vi "黑盾空调.vi"() -> ()   [LabVIEW 2016, in "环境动力监测库.lvlib" / "空调库.lvlib"]
uses:
  <vilib>/Utility/config.llb/NI_LVConfig.lvlib
  <vilib>/ptbypt/NI_PtbyPt.lvlib
panel:
  out "串口":string
  out "传感器状态":T1 {"系统模拟量量化数据"."电流A" format="%#.2g"}
  in  "查看型号":bool
  in  "重开串口":bool
  in  "校时":bool
  in  "设定参数":bool
  in  "遥控":bool
  out "获取设备厂家信息":T2
  out "仪器时间":timestamp
  out "系统参数":T3
  out "告警状态":T4
  out "写入缓冲区":string
  out "读取缓冲区":string
  out "读取选择":string(combo)
  out "通讯":bool
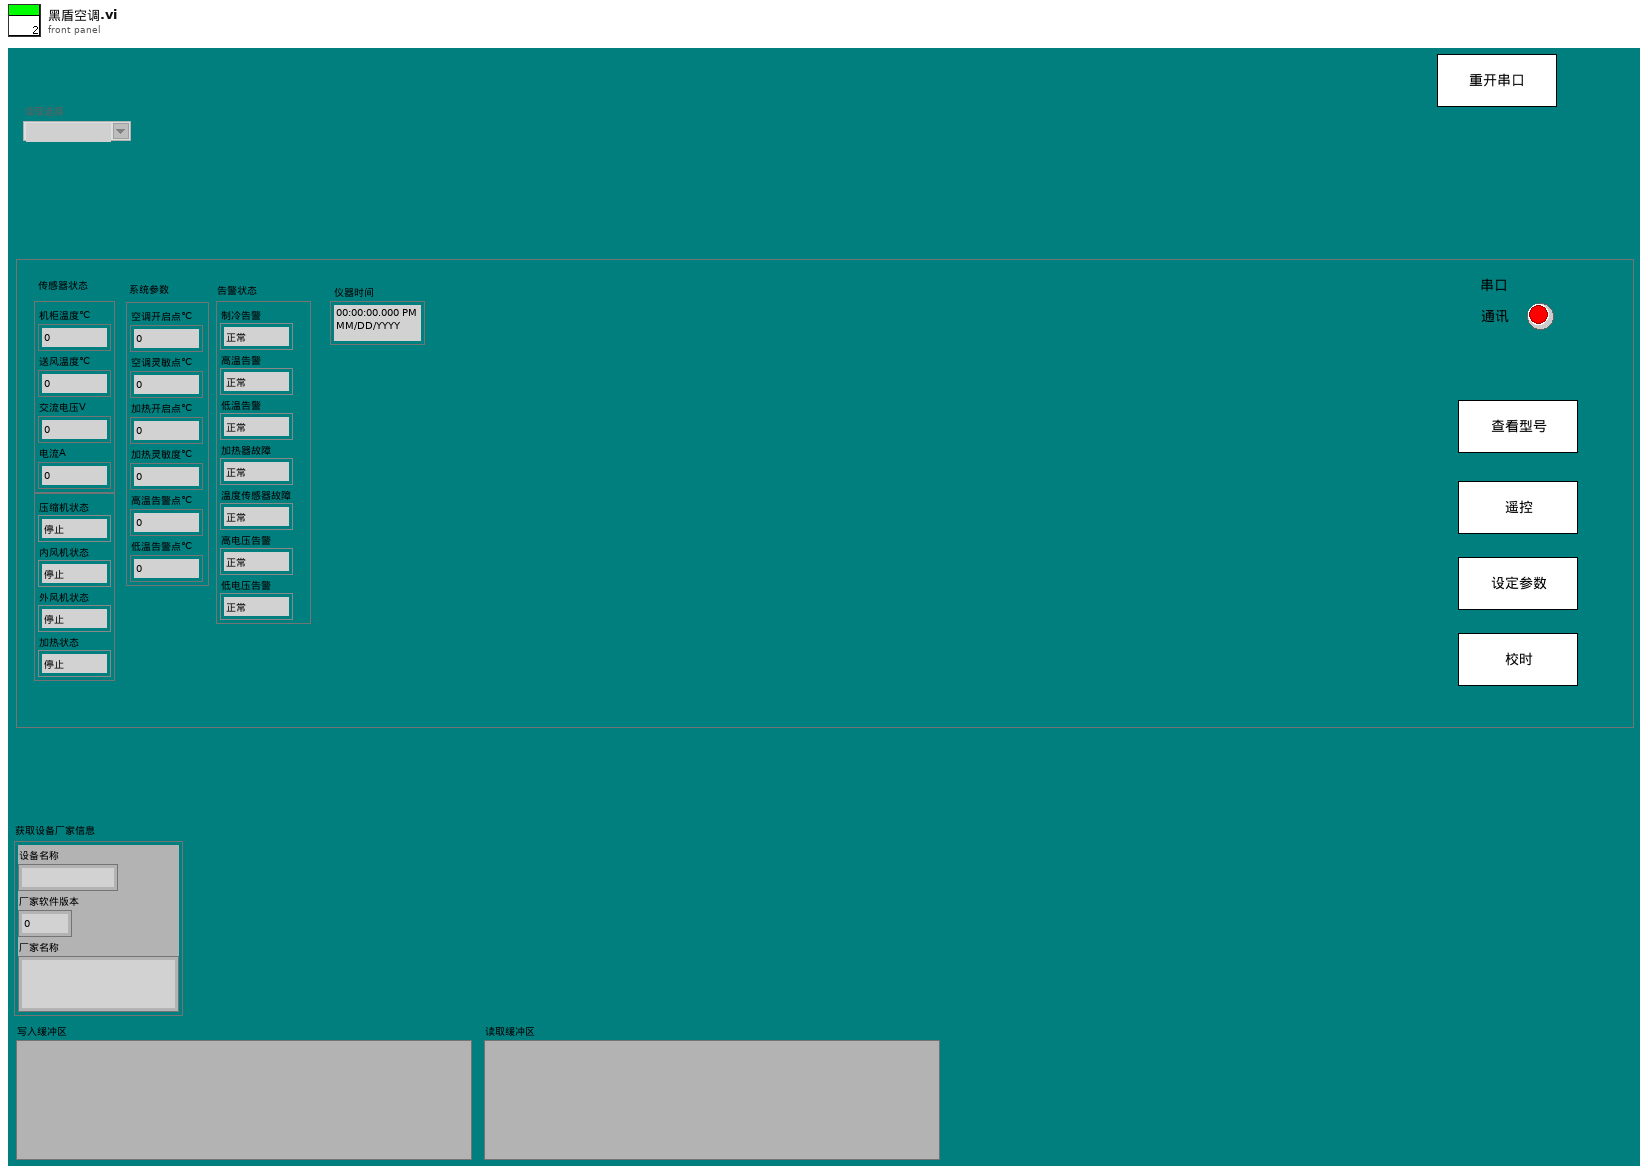
[diagram p1: front panel]
types:
  T1 = cluster{"系统模拟量量化数据":cluster{"机柜温度℃":sgl, "送风温度℃":sgl, "交流电压V":sgl, "电流A":sgl}, "开关量输入状态解析":cluster{"压缩机状态":enum16{"停止", "运行"}, "内风机状态":enum16{"停止", "运行"}, "外风机状态":enum16{"停止", "运行"}, "加热状态":enum16{"停止", "运行"}}}
  T2 = cluster{"设备名称":string, "厂家软件版本":u16, "厂家名称":string}
  T3 = cluster{"空调开启点℃":u16, "空调灵敏点℃":u16, "加热开启点℃":u16, "加热灵敏度℃":u16, "高温告警点℃":u16, "低温告警点℃":u16}
  T4 = cluster{"制冷告警":enum16{"正常", "告警"}, "高温告警":enum16{"正常", "告警"}, "低温告警":enum16{"正常", "告警"}, "加热器故障":enum16{"正常", "告警"}, "温度传感器故障":enum16{"正常", "告警"}, "高电压告警":enum16{"正常", "告警"}, "低电压告警":enum16{"正常", "告警"}, "预留":u16}
  T5 = cluster{"分支":enum16{"open", "read", "write", "close"}, "字符串":string}
  T6 = cluster{"分支":enum16{"open", "read", "write", "close"}, "读取选择":string}
  T7 = typedef "NI_LVConfig.lvlib/Config Data RefNum.ctl" = refnum<k1>
  T8 = cluster{"时间标识":timestamp, "设备":string, "日志信息":string}
  T9 = cluster{"漏水监测输出":cluster{"漏水监测告警":bool, "告警内容":string}, "门禁监测输出":cluster{"门禁监测告警":bool, "告警内容":string}, "温湿度监测输出":cluster{"温湿度监测告警":bool, "告警内容":string}, "烟雾监测输出":cluster{"烟雾监测告警":bool, "告警内容":string}, "空调监测输出":cluster{"空调监测告警":bool, "告警内容":string}, "自动重合闸输出":cluster{"自动重合闸告警":bool, "告警内容":string}, "红外入侵输出":cluster{"红外入侵告警":bool, "告警内容":string}, "振动输出":cluster{"振动告警":bool, "告警内容":string}, "UPS输出":cluster{"UPS告警":bool, "告警内容":string}, "蓄电池输出":cluster{"蓄电池告警":bool, "告警内容":string}, "GPS输出":cluster{"定位告警":bool, "告警内容":string}, "北斗输出":cluster{"定位告警":bool, "告警内容":string}, "气象输出":cluster{"气象告警":bool, "告警内容":string}}
  T10 = cluster{"温湿度":cluster{"温度:":sgl, "状态":bool, "湿度:":sgl}, "空调":cluster{"机柜温度:":sgl, "状态":bool, "压缩机:":enum16{"停止", "运行"}, "电加热:":enum16{"停止", "运行"}}, "排气扇":cluster{"排气扇:":enum16{"关闭", "打开"}}, "冰箱":cluster{"冰箱:":enum16{"关闭", "打开"}}}
  T11 = enum16{"获取模拟量量化数据（浮点数）", "获取模拟量量化数据（定点数）", "获取开关输入状态", "获取机柜空调告警状态", "遥控", "获取系统参数（浮点数）", "获取系统参数（定点数）", "设定系统参数（浮点数）", "设定系统参数（定点数）", "获取系统历史数据（浮点数）", "获取系统历史数据（定点数）", "获取历史告警", "获取监测模块时间", "设定监测模块时间", "获取通信协议版本号", "获取设备地址", "获取设备厂家信息", "设定设备地址（ADR）"}
  T12 = cluster{"分支":enum16{"open", "read", "write", "close"}, "连接的字符串":string}
  T13 = cluster{"机柜温度":sgl, "送风温度":sgl, "交流电压":sgl, "电流":sgl}
  T14 = cluster{"空调状态":enum16{"停止", "运行"}, "内风机状态":enum16{"停止", "运行"}, "外风机状态":enum16{"停止", "运行"}, "加热状态":enum16{"停止", "运行"}}
  T15 = cluster{"空调开启点":u16, "空调灵敏点":u16, "加热开启点":u16, "加热灵敏度":u16, "高温告警点":u16, "低温告警点":u16}
  T16 = enum16{"空调开机", "空调关机", "制冷开启", "制冷关闭", "制热开启", "制热关闭"}
  T17 = enum16{"空调开启点", "空调灵敏点", "加热开启点", "加热灵敏度", "高温告警点", "低温告警点"}
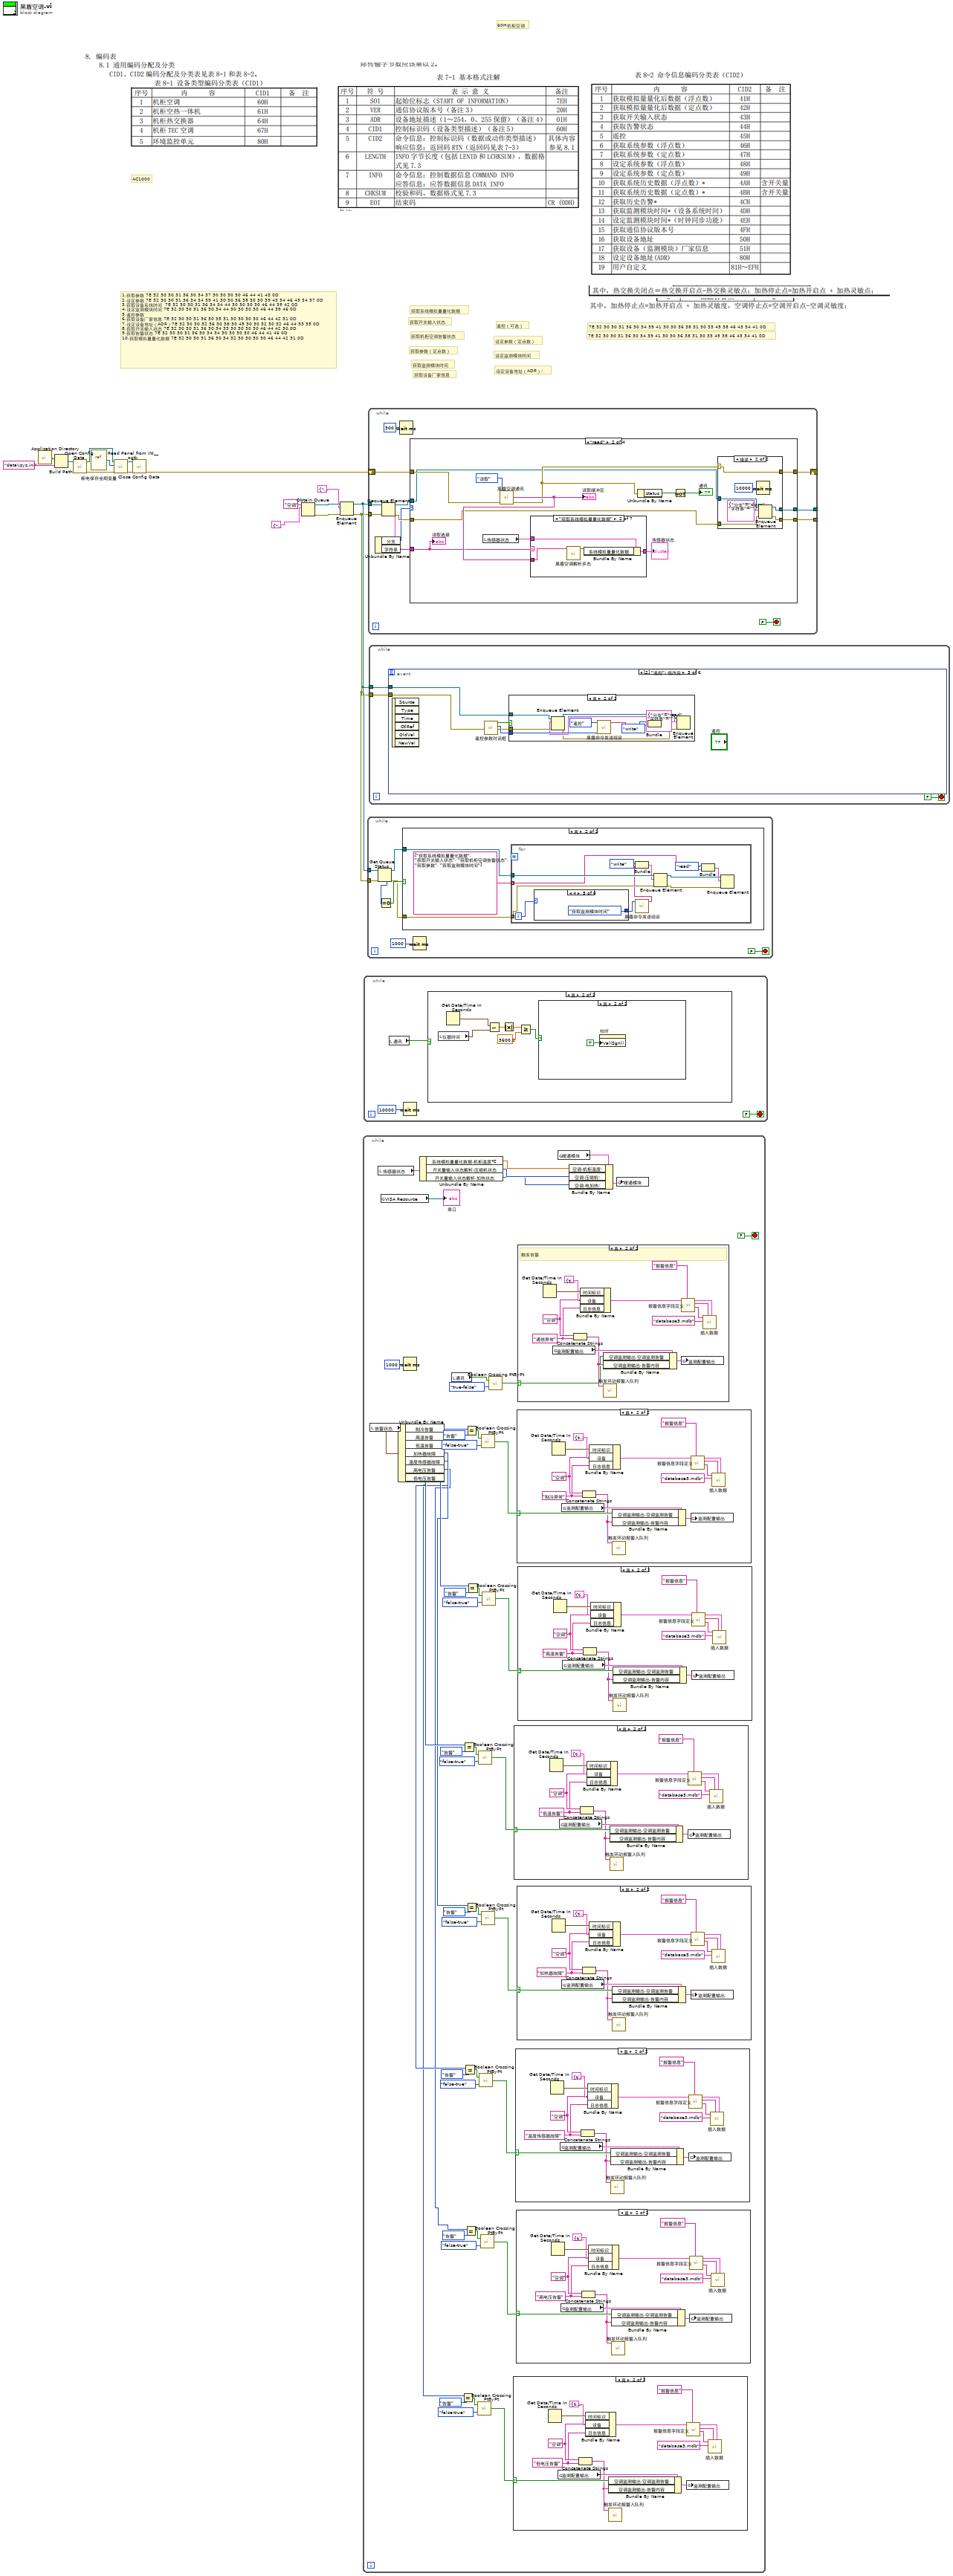
[diagram p0: block diagram]
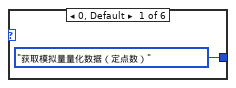
[diagram p13: hidden frame]
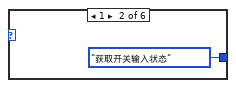
[diagram p14: hidden frame]
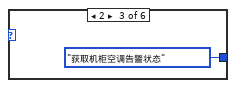
[diagram p15: hidden frame]
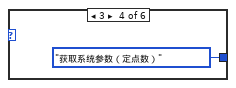
[diagram p16: hidden frame]
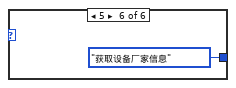
[diagram p17: hidden frame]
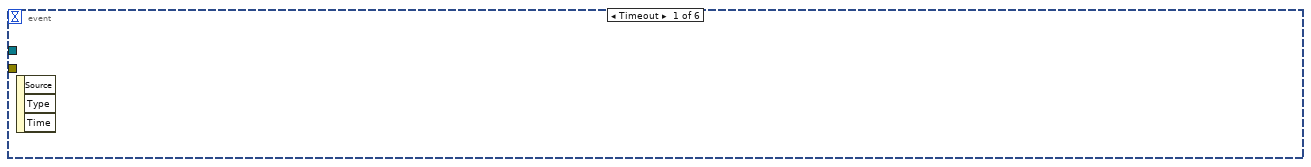
[diagram p18: hidden frame]
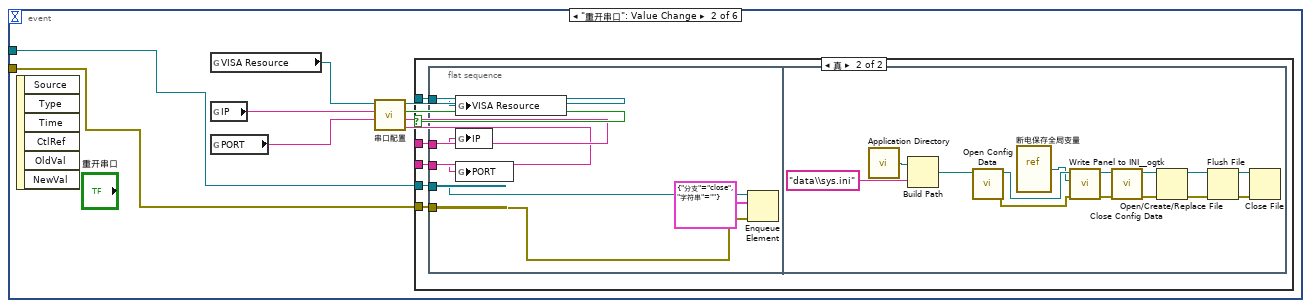
[diagram p19: hidden frame]
diagram:
  # "获取系统模拟量量化数据"
  # "设定设备地址（ADR）:"
  # "获取设备厂家信息"
  # "设定监测模块时间"
  # "获取监测模块时间"
  # "设定参数（定点数）"
  # "获取参数（定点数）"
  # "遥控（可选）"
  # "获取机柜空调告警状态"
  # "获取开关输入状态"
  # "7E 32 30 30 31 36 30 34 39 41 30 30 36 38 31 30 33 45 38 46 43 34 41 0D"
  # "7E 32 30 30 31 36 30 34 39 41 30 30 36 38 31 30 33 45 38 46 43 34 41 0D"
  # "60H机柜空调"
  # "AC1000"
  # "1.获取参数 7E 32 30 30 31 36 30 34 37 30 30 30 30 46 44 41 43 0D\n2.设定参数 7E 32 30 30 31 36 34 34 39 41 30 30 36 38 30 30 39 43 34 46 43 34 37 0D \n3.获取设备系统时间  7E 32 30 30 31 36 34 34 44 30 30 30 30 46 44 39 42 0D\n4.设定监测模块时间 7E 32 30 30 31 36 30 34 44 30 30 30 30 46 44 39 46 0D\n5.遥控参数\n6.获取设备厂家信息 7E 32 30 30 31 36 30 35 31 30 30 30 30 46 44 42 31 0D\n7.设定设备地址（ADR）7E 32 30 30 32 36 30 38 30 45 30 30 32 30 32 46 44 33 35 0D\n8.获取开关输入状态 7E 32 30 30 31 36 30 34 33 30 30 30 30 46 44 42 30 0D\n9.获取告警状态 7E 32 30 30 31 36 30 34 34 30 30 30 30 46 44 41 46 0D\n10.获取模拟量量化数据 7E 32 30 30 31 36 30 34 32 30 30 30 30 46 44 42 31 0D"
  n1 = call <vilib>:"Application Directory.vi"() -> ("Application Directory"=w16:path)
  n2 = Build Path(base path=w16, name or relative path="data\\sys.ini" ("名称或相对路径")) -> (appended path=w14:path)
  n3 = call <vilib>:"Open Config Data.vi"("configuration file path"=w14) -> ("error out"=w10:errorcluster, "refnum"=w13:T7)  [unwired: 8 in, 1 out]
  n4 = vi-ref "断电保存全局变量.vi"() -> (w12:refnum<vi>)
  n5 = call <userlib>:"Read Panel from INI__ogtk.vi"("error in (no error)"=w10, "VI ref"=w12, "refnum"=w13) -> ("error out"=w9:errorcluster, "refnum out"=w11:T7)  [unwired: 7 in]
  n6 = call <vilib>:"Close Config Data.vi"("error in (no error)"=w9, "refnum"=w11) -> ("error out"=w8:errorcluster)  [unwired: 8 in, 1 out]
  n7 = Obtain Queue(name (unnamed)="空调" ("名称（未命名）"), element data type=T5 {"分支"=enum."open", "字符串"="获取系统模拟量量化数据"}) -> (queue out=w6:refnum<queue>, error out=w5:errorcluster)  [unwired: 3 in, 1 out]
  n8 = Enqueue Element(queue=w6, element=T6 {"分支"=enum."open", "读取选择"="获取系统模拟量量化数据"}, error in (no error)=w5) -> (queue out=w4:refnum<queue>, error out=w3:errorcluster)  [unwired: 1 in, 1 out]
  n9 = while {
    stop <- FALSE stop-if-true
    n10 = local read "告警状态"() -> (w52:T4)
    n11 = local read "传感器状态"() -> (w59:T1)
    n12 = global read "断电保存全局变量.vi" "VISA Resource"() -> (→"串口":refnum<visa-resource-name>)
    n13 = Unbundle By Name(w52) -> ("制冷告警"=w51:enum16{"正常", "告警"}, "高温告警"=w42:enum16{"正常", "告警"}, "低温告警"=w37:enum16{"正常", "告警"}, "加热器故障"=w32:enum16{"正常", "告警"}, "温度传感器故障"=w27:enum16{"正常", "告警"}, "高电压告警"=w18:enum16{"正常", "告警"}, "低电压告警"=w17:enum16{"正常", "告警"})
    n14 = Wait (ms)(milliseconds to wait=u32 1000 ("等待时间（毫秒）")) -> ()  [unwired: 1 out]
    n15 = Unbundle By Name(w59) -> ("系统模拟量量化数据.机柜温度℃"=w58:sgl, "开关量输入状态解析.压缩机状态"=w57:enum16{"停止", "运行"}, "开关量输入状态解析.加热状态"=w56:enum16{"停止", "运行"})
    n16 = local read "通讯"() -> (w53:bool)
    n17 = Equal?(x=w17, y=enum16{"正常", "告警"}."告警") -> (x = y?=w20:bool)
    n18 = Equal?(x=w37, y=enum16{"正常", "告警"}."告警") -> (x = y?=w39:bool)
    n19 = Equal?(x=w27, y=enum16{"正常", "告警"}."告警") -> (x = y?=w29:bool)
    n20 = Equal?(x=w18, y=enum16{"正常", "告警"}."告警") -> (x = y?=w24:bool)
    n21 = Equal?(x=w51, y=enum16{"正常", "告警"}."告警") -> (x = y?=w48:bool)
    n22 = Equal?(x=w32, y=enum16{"正常", "告警"}."告警") -> (x = y?=w34:bool)
    n23 = Equal?(x=w42, y=enum16{"正常", "告警"}."告警") -> (x = y?=w44:bool)
    n24 = call <vilib>:"Boolean Crossing PtByPt.vi"("direction"=enum16{"either", "false-true", "true-false"}."false-true", "input"=w20) -> ("crossing"=w19:bool)  [unwired: 1 in]
    n25 = call <vilib>:"Boolean Crossing PtByPt.vi"("direction"=enum16{"either", "false-true", "true-false"}."false-true", "input"=w39) -> ("crossing"=w38:bool)  [unwired: 1 in]
    n26 = call <vilib>:"Boolean Crossing PtByPt.vi"("direction"=enum16{"either", "false-true", "true-false"}."false-true", "input"=w29) -> ("crossing"=w28:bool)  [unwired: 1 in]
    n27 = call <vilib>:"Boolean Crossing PtByPt.vi"("direction"=enum16{"either", "false-true", "true-false"}."false-true", "input"=w24) -> ("crossing"=w23:bool)  [unwired: 1 in]
    n28 = call <vilib>:"Boolean Crossing PtByPt.vi"("direction"=enum16{"either", "false-true", "true-false"}."false-true", "input"=w48) -> ("crossing"=w47:bool)  [unwired: 1 in]
    n29 = call <vilib>:"Boolean Crossing PtByPt.vi"("direction"=enum16{"either", "false-true", "true-false"}."false-true", "input"=w34) -> ("crossing"=w33:bool)  [unwired: 1 in]
    n30 = call <vilib>:"Boolean Crossing PtByPt.vi"("direction"=enum16{"either", "false-true", "true-false"}."false-true", "input"=w44) -> ("crossing"=w43:bool)  [unwired: 1 in]
    n31 = call <vilib>:"Boolean Crossing PtByPt.vi"("direction"=enum16{"either", "false-true", "true-false"}."true-false", "input"=w53) -> ("crossing"=w54:bool)  [unwired: 1 in]
    n32 = case shown="真" w19 {
      selector: w19 -> [_ w68]
      frame False {
      }
      frame True {
        w66 = "低电压告警" ("日志信息")
        w67 = "空调" ("设备")
        n33 = Get Date/Time In Seconds() -> (seconds since 1Jan1904=w78:timestamp)
        n34 = global read "断电保存全局变量.vi" "监测配置输出"() -> (w69:T9)
        n35 = Concatenate Strings(w67, w66) -> (w65:string)
        n36 = Bundle By Name(cluster=T8 {"时间标识"=timestamp(0 s since 1904-01-01), "设备"="", "日志信息"=""} ("data in"), "时间标识"=w78, "设备"=w67, "日志信息"=w66) -> (w77:T8)
        n37 = Bundle By Name(cluster=w69, "空调监测输出.空调监测告警"=w68, "空调监测输出.告警内容"=w65) -> (w70:T9)
        n38 = call "触发环动报警入队列.vi"("报警内容"=w65) -> ()  [unwired: 11 in]
        n39 = call "报警信息字段定义.vi"("table输入"="报警信息", "data in"=w77) -> ("table输出"=w73:string, "columns"=w72:string[], "data out"=w71:T8)  [unwired: 7 in]
        n40 = global write "断电保存全局变量.vi" "监测配置输出"(w70) -> ()
        n41 = call "插入数据.vi"("data"=w71, "columns"=w72, "database"="database3.mdb", "table"=w73) -> ()  [unwired: 7 in, 1 out]
      }
    }
    n42 = case shown="真" w38 {
      selector: w38 -> [_ w124]
      frame False {
      }
      frame True {
        w122 = "低温告警" ("日志信息")
        w123 = "空调" ("设备")
        n43 = Get Date/Time In Seconds() -> (seconds since 1Jan1904=w134:timestamp)
        n44 = global read "断电保存全局变量.vi" "监测配置输出"() -> (w125:T9)
        n45 = Concatenate Strings(w123, w122) -> (w121:string)
        n46 = Bundle By Name(cluster=T8 {"时间标识"=timestamp(0 s since 1904-01-01), "设备"="", "日志信息"=""} ("data in"), "时间标识"=w134, "设备"=w123, "日志信息"=w122) -> (w133:T8)
        n47 = Bundle By Name(cluster=w125, "空调监测输出.空调监测告警"=w124, "空调监测输出.告警内容"=w121) -> (w126:T9)
        n48 = call "触发环动报警入队列.vi"("报警内容"=w121) -> ()  [unwired: 11 in]
        n49 = call "报警信息字段定义.vi"("table输入"="报警信息", "data in"=w133) -> ("table输出"=w129:string, "columns"=w128:string[], "data out"=w127:T8)  [unwired: 7 in]
        n50 = global write "断电保存全局变量.vi" "监测配置输出"(w126) -> ()
        n51 = call "插入数据.vi"("data"=w127, "columns"=w128, "database"="database3.mdb", "table"=w129) -> ()  [unwired: 7 in, 1 out]
      }
    }
    n52 = case shown="真" w28 {
      selector: w28 -> [_ w96]
      frame False {
      }
      frame True {
        w94 = "温度传感器故障" ("日志信息")
        w95 = "空调" ("设备")
        n53 = Get Date/Time In Seconds() -> (seconds since 1Jan1904=w106:timestamp)
        n54 = global read "断电保存全局变量.vi" "监测配置输出"() -> (w97:T9)
        n55 = Concatenate Strings(w95, w94) -> (w93:string)
        n56 = Bundle By Name(cluster=T8 {"时间标识"=timestamp(0 s since 1904-01-01), "设备"="", "日志信息"=""} ("data in"), "时间标识"=w106, "设备"=w95, "日志信息"=w94) -> (w105:T8)
        n57 = Bundle By Name(cluster=w97, "空调监测输出.空调监测告警"=w96, "空调监测输出.告警内容"=w93) -> (w98:T9)
        n58 = call "触发环动报警入队列.vi"("报警内容"=w93) -> ()  [unwired: 11 in]
        n59 = call "报警信息字段定义.vi"("table输入"="报警信息", "data in"=w105) -> ("table输出"=w101:string, "columns"=w100:string[], "data out"=w99:T8)  [unwired: 7 in]
        n60 = global write "断电保存全局变量.vi" "监测配置输出"(w98) -> ()
        n61 = call "插入数据.vi"("data"=w99, "columns"=w100, "database"="database3.mdb", "table"=w101) -> ()  [unwired: 7 in, 1 out]
      }
    }
    n62 = case shown="真" w23 {
      selector: w23 -> [_ w82]
      frame False {
      }
      frame True {
        w80 = "高电压告警" ("日志信息")
        w81 = "空调" ("设备")
        n63 = Get Date/Time In Seconds() -> (seconds since 1Jan1904=w92:timestamp)
        n64 = global read "断电保存全局变量.vi" "监测配置输出"() -> (w83:T9)
        n65 = Concatenate Strings(w81, w80) -> (w79:string)
        n66 = Bundle By Name(cluster=T8 {"时间标识"=timestamp(0 s since 1904-01-01), "设备"="", "日志信息"=""} ("data in"), "时间标识"=w92, "设备"=w81, "日志信息"=w80) -> (w91:T8)
        n67 = Bundle By Name(cluster=w83, "空调监测输出.空调监测告警"=w82, "空调监测输出.告警内容"=w79) -> (w84:T9)
        n68 = call "触发环动报警入队列.vi"("报警内容"=w79) -> ()  [unwired: 11 in]
        n69 = call "报警信息字段定义.vi"("table输入"="报警信息", "data in"=w91) -> ("table输出"=w87:string, "columns"=w86:string[], "data out"=w85:T8)  [unwired: 7 in]
        n70 = global write "断电保存全局变量.vi" "监测配置输出"(w84) -> ()
        n71 = call "插入数据.vi"("data"=w85, "columns"=w86, "database"="database3.mdb", "table"=w87) -> ()  [unwired: 7 in, 1 out]
      }
    }
    n72 = case shown="真" w47 {
      selector: w47 -> [_ w152]
      frame False {
      }
      frame True {
        w150 = "制冷异常" ("日志信息")
        w151 = "空调" ("设备")
        n73 = Get Date/Time In Seconds() -> (seconds since 1Jan1904=w162:timestamp)
        n74 = global read "断电保存全局变量.vi" "监测配置输出"() -> (w153:T9)
        n75 = Concatenate Strings(w151, w150) -> (w149:string)
        n76 = Bundle By Name(cluster=T8 {"时间标识"=timestamp(0 s since 1904-01-01), "设备"="", "日志信息"=""} ("data in"), "时间标识"=w162, "设备"=w151, "日志信息"=w150) -> (w161:T8)
        n77 = Bundle By Name(cluster=w153, "空调监测输出.空调监测告警"=w152, "空调监测输出.告警内容"=w149) -> (w154:T9)
        n78 = call "触发环动报警入队列.vi"("报警内容"=w149) -> ()  [unwired: 11 in]
        n79 = call "报警信息字段定义.vi"("table输入"="报警信息", "data in"=w161) -> ("table输出"=w157:string, "columns"=w156:string[], "data out"=w155:T8)  [unwired: 7 in]
        n80 = global write "断电保存全局变量.vi" "监测配置输出"(w154) -> ()
        n81 = call "插入数据.vi"("data"=w155, "columns"=w156, "database"="database3.mdb", "table"=w157) -> ()  [unwired: 7 in, 1 out]
      }
    }
    n82 = case shown="真" w33 {
      selector: w33 -> [_ w110]
      frame False {
      }
      frame True {
        w108 = "加热器故障" ("日志信息")
        w109 = "空调" ("设备")
        n83 = Get Date/Time In Seconds() -> (seconds since 1Jan1904=w120:timestamp)
        n84 = global read "断电保存全局变量.vi" "监测配置输出"() -> (w111:T9)
        n85 = Concatenate Strings(w109, w108) -> (w107:string)
        n86 = Bundle By Name(cluster=T8 {"时间标识"=timestamp(0 s since 1904-01-01), "设备"="", "日志信息"=""} ("data in"), "时间标识"=w120, "设备"=w109, "日志信息"=w108) -> (w119:T8)
        n87 = Bundle By Name(cluster=w111, "空调监测输出.空调监测告警"=w110, "空调监测输出.告警内容"=w107) -> (w112:T9)
        n88 = call "触发环动报警入队列.vi"("报警内容"=w107) -> ()  [unwired: 11 in]
        n89 = call "报警信息字段定义.vi"("table输入"="报警信息", "data in"=w119) -> ("table输出"=w115:string, "columns"=w114:string[], "data out"=w113:T8)  [unwired: 7 in]
        n90 = global write "断电保存全局变量.vi" "监测配置输出"(w112) -> ()
        n91 = call "插入数据.vi"("data"=w113, "columns"=w114, "database"="database3.mdb", "table"=w115) -> ()  [unwired: 7 in, 1 out]
      }
    }
    n92 = case shown="真" w54 {
      selector: w54 -> [_ w163]
      frame False {
      }
      frame True {
        w165 = "通信异常" ("日志信息")
        w166 = "空调" ("设备")
        # "触发告警"
        n93 = Get Date/Time In Seconds() -> (seconds since 1Jan1904=w176:timestamp)
        n94 = global read "断电保存全局变量.vi" "监测配置输出"() -> (w167:T9)
        n95 = Concatenate Strings(w166, w165) -> (w164:string)
        n96 = Bundle By Name(cluster=T8 {"时间标识"=timestamp(0 s since 1904-01-01), "设备"="", "日志信息"=""} ("data in"), "时间标识"=w176, "设备"=w166, "日志信息"=w165) -> (w175:T8)
        n97 = Bundle By Name(cluster=w167, "空调监测输出.空调监测告警"=w163, "空调监测输出.告警内容"=w164) -> (w168:T9)
        n98 = call "触发环动报警入队列.vi"("报警内容"=w164) -> ()  [unwired: 11 in]
        n99 = call "报警信息字段定义.vi"("table输入"="报警信息", "data in"=w175) -> ("table输出"=w171:string, "columns"=w170:string[], "data out"=w169:T8)  [unwired: 7 in]
        n100 = global write "断电保存全局变量.vi" "监测配置输出"(w168) -> ()
        n101 = call "插入数据.vi"("data"=w169, "columns"=w170, "database"="database3.mdb", "table"=w171) -> ()  [unwired: 7 in, 1 out]
      }
    }
    n102 = case shown="真" w43 {
      selector: w43 -> [_ w138]
      frame False {
      }
      frame True {
        w136 = "高温告警" ("日志信息")
        w137 = "空调" ("设备")
        n103 = Get Date/Time In Seconds() -> (seconds since 1Jan1904=w148:timestamp)
        n104 = global read "断电保存全局变量.vi" "监测配置输出"() -> (w139:T9)
        n105 = Concatenate Strings(w137, w136) -> (w135:string)
        n106 = Bundle By Name(cluster=T8 {"时间标识"=timestamp(0 s since 1904-01-01), "设备"="", "日志信息"=""} ("data in"), "时间标识"=w148, "设备"=w137, "日志信息"=w136) -> (w147:T8)
        n107 = Bundle By Name(cluster=w139, "空调监测输出.空调监测告警"=w138, "空调监测输出.告警内容"=w135) -> (w140:T9)
        n108 = call "触发环动报警入队列.vi"("报警内容"=w135) -> ()  [unwired: 11 in]
        n109 = call "报警信息字段定义.vi"("table输入"="报警信息", "data in"=w147) -> ("table输出"=w143:string, "columns"=w142:string[], "data out"=w141:T8)  [unwired: 7 in]
        n110 = global write "断电保存全局变量.vi" "监测配置输出"(w140) -> ()
        n111 = call "插入数据.vi"("data"=w141, "columns"=w142, "database"="database3.mdb", "table"=w143) -> ()  [unwired: 7 in, 1 out]
      }
    }
    n112 = global read "内部交互全局变量.vi" "暖通模块"() -> (w61:T10)
    n113 = Bundle By Name(cluster=w61, "空调.机柜温度:"=w58, "空调.压缩机:"=w57, "空调.电加热:"=w56) -> (w60:T10)
    n114 = global write "内部交互全局变量.vi" "暖通模块"(w60) -> ()
  }
  n115 = while {
    stop <- FALSE stop-if-true
    n116 = local read "通讯"() -> (w178:bool)
    n117 = Wait (ms)(milliseconds to wait=u32 10000 ("等待时间（毫秒）")) -> ()  [unwired: 1 out]
    n118 = case shown="真" w178 {
      frame False {
      }
      frame True {
        n119 = local read "仪器时间"() -> (w184:timestamp)
        n120 = Get Date/Time In Seconds() -> (seconds since 1Jan1904=w185:timestamp)
        n121 = Subtract(x=w185, y=w184) -> (x-y=w183:dbl)
        n122 = Absolute Value(x=w183) -> (abs(x)=w182:dbl)
        n123 = Greater Or Equal?(x=w182, y=3600.0) -> (x >= y?=w180:bool)
        n124 = case shown="真" w180 {
          frame False {
          }
          frame True {
            n125 = property on="校时" class="Bool"("Val(Sgnl)"=TRUE) -> ()  [unwired: 2 in, 2 out]
          }
        }
      }
    }
  }
  n126 = while {
    tunnel: w4 -> [w193]
    tunnel: w3 -> [w192]
    stop <- FALSE stop-if-true
    n127 = Get Queue Status(queue=w193, error in (no error)=w192) -> (queue out=w189:refnum<queue>, error out=w188:errorcluster, # elements in queue=w191:i32)  [unwired: 1 in, 5 out]
    n128 = Equal To 0?(x=w191) -> (x = 0?=w190:bool)
    n129 = case shown="真" w190 {
      tunnel: w189 -> [_ w196]
      tunnel: w188 -> [_ w195]
      frame False {
      }
      frame True {
        n130 = for {
          tunnel: string[] ["获取系统模拟量量化数据", "获取开关输入状态", "获取机柜空调告警状态", "获取参数", "获取监测模块时间"] -> [w199] mode=indexing
          tunnel: w196 -> [w209]
          tunnel: w195 -> [w208]
          i -> [w207]
          n131 = case shown="4" w207 {
            tunnel: [T11."获取模拟量量化数据（定点数）" ("CID2枚举") T11."获取开关输入状态" ("CID2枚举") T11."获取机柜空调告警状态" ("CID2枚举") T11."获取系统参数（定点数）" ("CID2枚举") T11."获取监测模块时间" ("CID2枚举") T11."获取设备厂家信息" ("CID2枚举")] -> w206
            frame 0, Default {
            }
            frame 1 {
            }
            frame 2 {
            }
            frame 3 {
            }
            frame 4 {
            }
            frame 5 {
            }
          }
          n132 = call "黑盾命令发送组合.vi"("CID2枚举"=w206) -> ("连接的字符串"=w204:string)  [unwired: 10 in]
          n133 = Bundle("分支"=enum16{"open", "read", "write", "close"}."write", "连接的字符串"=w204) -> (w203:T12)  [unwired: 1 in]
          n134 = Enqueue Element(queue=w209, element=w203, error in (no error)=w208) -> (queue out=w201:refnum<queue>, error out=w200:errorcluster)  [unwired: 1 in, 1 out]
          n135 = Bundle("分支"=enum16{"open", "read", "write", "close"}."read", "读取选择"=w199) -> (w198:T6)  [unwired: 1 in]
          n136 = Enqueue Element(queue=w201, element=w198, error in (no error)=w200) -> ()  [unwired: 1 in, 3 out]
        }
      }
    }
    n137 = Wait (ms)(milliseconds to wait=u32 1000 ("等待时间（毫秒）")) -> ()  [unwired: 1 out]
  }
  n138 = while {
    tunnel: w4 -> [w226]
    tunnel: w3 -> [w225]
    shift-right: [w224] -> _
    shift-left: w8 -> [w223]
    tunnel: [w220] -> _
    tunnel: [w219] -> _
    stop <- FALSE stop-if-true
    n139 = Dequeue Element(queue=w226, error in (no error)=w225) -> (queue out=w222:refnum<queue>, element=w218:T5, error out=w221:errorcluster)  [unwired: 1 in, 1 out]
    n140 = Unbundle By Name(w218) -> ("分支"=w217:enum16{"open", "read", "write", "close"}, "字符串"=w216:string)
    n141 = Wait (ms)(milliseconds to wait=u32 300 ("等待时间（毫秒）")) -> ()  [unwired: 1 out]
    n142 = case shown="\"read\"" w217 {
      tunnel: [w231 w235 w282 w290] -> w224
      tunnel: w223 -> [_ w246 w283 w291]
      tunnel: w222 -> [w230 w239 w280 w289]
      tunnel: w221 -> [w229 w237 w279 w288]
      tunnel: [w230 w238 w280 w286] -> w220
      tunnel: [w229 w236 w279 w285] -> w219
      tunnel: w216 -> [_ w244 w281 _]
      frame "open", Default {
        n143 = global read "断电保存全局变量.vi" "VISA Resource"() -> (w232:refnum<visa-resource-name>)
        n144 = call "黑盾空调通讯.vi"("VISA resource name"=w232, "功能输入"=enum16{"打开串口", "写入", "读取", "关闭串口"}."打开串口") -> ("error out"=w231:errorcluster)  [unwired: 7 in, 2 out]
      }
      frame "read" {
        n145 = local read "传感器状态"() -> (w242:T1)
        n146 = call "黑盾空调通讯.vi"("error in (no error)"=w246, "功能输入"=enum16{"打开串口", "写入", "读取", "关闭串口"}."读取") -> ("error out"=w240:errorcluster, "读取缓冲区"=w245:string)  [unwired: 7 in, 1 out]
        "读取缓冲区" <- w245
        n147 = case shown="\"获取系统模拟量量化数据\"" w244 {
          tunnel: w245 -> [_ w262 w266 w269 w272 w275 w278]
          tunnel: w242 -> [w258 w261 w265 w267 w270 w273 w276]
          tunnel: [w258 w259 w263 w267 w270 w273 w276] -> w241
          frame "假", Default {
          }
          frame "获取系统模拟量量化数据" {
            n148 = call-poly "黑盾空调解析多态.vi"("输入字符串"=w262) -> ("系统模拟量量化数据"=w260:T13)  [unwired: 10 in]
            n149 = Bundle By Name(cluster=w261, "系统模拟量量化数据"=w260) -> (w259:T1)
          }
          frame "获取开关输入状态" {
            n150 = call-poly "黑盾空调解析多态.vi"("输入字符串"=w266) -> ("开关量输入状态解析"=w264:T14)  [unwired: 10 in]
            n151 = Bundle By Name(cluster=w265, "开关量输入状态解析"=w264) -> (w263:T1)
          }
          frame "获取机柜空调告警状态" {
            n152 = call-poly "黑盾空调解析多态.vi"("输入字符串"=w269) -> ("机柜空调告警状态"=→"告警状态":T4)  [unwired: 10 in]
          }
          frame "获取参数" {
            n153 = call-poly "黑盾空调解析多态.vi"("输入字符串"=w272) -> ("获取参数(定点数)"=→"系统参数":T15)  [unwired: 10 in]
          }
          frame "获取监测模块时间" {
            n154 = call-poly "黑盾空调解析多态.vi"("输入字符串"=w275) -> ("时间标识"=→"仪器时间":timestamp)  [unwired: 10 in]
          }
          frame "获取设备厂家信息" {
            n155 = call-poly "黑盾空调解析多态.vi"("输入字符串"=w278) -> ("获取设备厂家信息"=→"获取设备厂家信息":T2)  [unwired: 10 in]
          }
        }
        "传感器状态" <- w241
        n156 = Unbundle By Name(w240) -> ("status"=w243:bool)
        n157 = Not(x=w243) -> (.not. x?=→"通讯":bool)
        n158 = case shown="错误" w240 {
          selector: w240 -> [w250 w252]
          tunnel: w239 -> [w249 w256]
          tunnel: [w249 w255] -> w238
          tunnel: w237 -> [w248 w254]
          tunnel: [w248 w253] -> w236
          tunnel: [w250 w252] -> w235
          frame No Error {
          }
          frame Error {
            n159 = Wait (ms)(milliseconds to wait=u32 10000 ("等待时间（毫秒）")) -> ()  [unwired: 1 out]
            n160 = Enqueue Element(queue=w256, element=T5 {"分支"=enum."close", "字符串"=""} ("元素"), error in (no error)=w254) -> (queue out=w255:refnum<queue>, error out=w253:errorcluster)  [unwired: 1 in, 1 out]
          }
        }
        "读取选择" <- w244
      }
      frame "write" {
        n161 = call "黑盾空调通讯.vi"("error in (no error)"=w283, "写入缓冲区"=w281, "功能输入"=enum16{"打开串口", "写入", "读取", "关闭串口"}."写入") -> ("error out"=w282:errorcluster)  [unwired: 6 in, 2 out]
        "写入缓冲区" <- w281
      }
      frame "close" {
        n162 = call "黑盾空调通讯.vi"("error in (no error)"=w291, "功能输入"=enum16{"打开串口", "写入", "读取", "关闭串口"}."关闭串口") -> ("error out"=w290:errorcluster)  [unwired: 7 in, 2 out]
        n163 = Enqueue Element(queue=w289, element=T5 {"分支"=enum."open", "字符串"=""} ("元素"), error in (no error)=w288) -> (queue out=w286:refnum<queue>, error out=w285:errorcluster)  [unwired: 1 in, 1 out]
      }
    }
  }
  n164 = while {
    tunnel: w4 -> [w294]
    tunnel: w3 -> [w293]
    stop <- FALSE stop-if-true
    n165 = event shown="[2] \"遥控\": 值改变" {
      selector: _ -> [_ _ _ _ _ _]
      dyn-events: _ -> [_ _ _ _ _ _]
      timeout: _ -> [_ _ _ _ _ _]
      tunnel: w294 -> [_ w297 w330 w349 w369 _]
      tunnel: w293 -> [_ w296 w331 w348 w368 _]
      event Timeout {
        n166 = event-data() -> ()  [unwired: 1 in, 3 out]
      }
      event "重开串口": Value Change {
        n167 = event-data() -> ()  [unwired: 1 in, 6 out]
        n168 = global read "断电保存全局变量.vi" "VISA Resource"() -> (w304:refnum<visa-resource-name>)
        n169 = global read "断电保存全局变量.vi" "IP"() -> (w299:string)
        n170 = global read "断电保存全局变量.vi" "PORT"() -> (w298:string)
        n171 = call "串口配置.vi"("PORT"=w298, "IP"=w299, "请选择串口:"=w304) -> ("PORT 2"=w300:string, "IP 2"=w301:string, "确认 2"=w302:bool, "VISA资源名称 2"=w303:refnum<visa-resource-name>)  [unwired: 5 in]
        n172 = case shown="真" w302 {
          tunnel: w303 -> [_ w307]
          tunnel: w297 -> [_ w309]
          tunnel: w296 -> [_ w308]
          tunnel: w301 -> [_ w306]
          tunnel: w300 -> [_ w305]
          frame False {
          }
          frame True {
            n173 = flat-sequence {
              tunnel: w309 -> [w315]
              tunnel: w308 -> [w314]
              tunnel: w307 -> [w313]
              tunnel: w306 -> [w312]
              tunnel: w305 -> [w311]
              frame #0 {
                n174 = global write "断电保存全局变量.vi" "VISA Resource"(w313) -> ()
                n175 = global write "断电保存全局变量.vi" "IP"(w312) -> ()
                n176 = global write "断电保存全局变量.vi" "PORT"(w311) -> ()
                n177 = Enqueue Element(queue=w315, element=T5 {"分支"=enum."close", "字符串"=""} ("元素"), error in (no error)=w314) -> ()  [unwired: 1 in, 3 out]
              }
              frame #1 {
                n178 = call <vilib>:"Application Directory.vi"() -> ("Application Directory"=w328:path)
                n179 = Build Path(base path=w328, name or relative path="data\\sys.ini" ("名称或相对路径")) -> (appended path=w327:path)
                n180 = call <vilib>:"Open Config Data.vi"("configuration file path"=w327) -> ("error out"=w323:errorcluster, "refnum"=w326:T7)  [unwired: 8 in, 1 out]
                n181 = vi-ref "断电保存全局变量.vi"() -> (w325:refnum<vi>)
                n182 = call <userlib>:"Write Panel to INI__ogtk.vi"("error in (no error)"=w323, "VI ref"=w325, "refnum"=w326) -> ("error out"=w322:errorcluster, "refnum out"=w324:T7)  [unwired: 7 in]
                n183 = call <vilib>:"Close Config Data.vi"("error in (no error)"=w322, "refnum"=w324) -> ("error out"=w317:errorcluster, "file path"=w316:path)  [unwired: 8 in]
                n184 = Open/Create/Replace File(file path (use dialog)=w316, error in=w317) -> (refnum out=w320:refnum<file>, error out=w321:errorcluster)  [unwired: 4 in, 1 out]
                n185 = Flush File(refnum=w320, error in=w321) -> (refnum out=w319:refnum<file>, error out=w318:errorcluster)
                n186 = Close File(refnum=w319, error in=w318) -> ()  [unwired: 2 out]
              }
            }
          }
        }
      }
      event "遥控": Value Change {
        n187 = event-data() -> ()  [unwired: 1 in, 6 out]
        n188 = call "遥控参数对话框.vi"() -> ("遥控参数选择输出"=w332:T16, "确定?"=w333:bool)  [unwired: 10 in]
        n189 = case shown="真" w333 {
          tunnel: w332 -> [_ w342]
          tunnel: w331 -> [_ w341]
          tunnel: w330 -> [_ w340]
          frame False {
          }
          frame True {
            n190 = call "黑盾命令发送组合.vi"("遥控参数选择"=w342, "CID2枚举"=T11."遥控") -> ("连接的字符串"=w338:string)  [unwired: 9 in]
            n191 = Bundle("分支"=enum16{"open", "read", "write", "close"}."write", "连接的字符串"=w338) -> (w337:T12)  [unwired: 1 in]
            n192 = Enqueue Element(queue=w340, element=w337, error in (no error)=w341) -> (queue out=w336:refnum<queue>, error out=w335:errorcluster)  [unwired: 1 in, 1 out]
            n193 = Enqueue Element(queue=w336, element=T5 {"分支"=enum."read", "字符串"=""} ("元素"), error in (no error)=w335) -> ()  [unwired: 1 in, 3 out]
          }
        }
      }
      event "设定参数": Value Change {
        n194 = event-data() -> ()  [unwired: 1 in, 6 out]
        n195 = local read "系统参数"() -> (w344:T3)
        n196 = call "设定参数对话框.vi"("获取参数(定点数)"=w344) -> ("参数 2"=w345:u16, "设定参数（定点数）选择 2"=w346:T17, "确定?"=w347:bool)  [unwired: 8 in]
        n197 = case shown="真" w347 {
          tunnel: w348 -> [_ w359]
          tunnel: w349 -> [_ w358]
          tunnel: w346 -> [_ w357]
          tunnel: w345 -> [_ w356]
          frame False {
          }
          frame True {
            n198 = call "黑盾命令发送组合.vi"("参数"=w356, "设定参数（定点数）选择"=w357, "CID2枚举"=T11."设定系统参数（定点数）") -> ("连接的字符串"=w354:string)  [unwired: 8 in]
            n199 = Bundle("分支"=enum16{"open", "read", "write", "close"}."write", "连接的字符串"=w354) -> (w353:T12)  [unwired: 1 in]
            n200 = Enqueue Element(queue=w358, element=w353, error in (no error)=w359) -> (queue out=w352:refnum<queue>, error out=w351:errorcluster)  [unwired: 1 in, 1 out]
            n201 = Enqueue Element(queue=w352, element=T5 {"分支"=enum."read", "字符串"=""} ("元素"), error in (no error)=w351) -> ()  [unwired: 1 in, 3 out]
          }
        }
      }
      event "校时": Value Change {
        n202 = event-data() -> ()  [unwired: 1 in, 6 out]
        n203 = call "黑盾命令发送组合.vi"("CID2枚举"=T11."设定监测模块时间") -> ("连接的字符串"=w365:string)  [unwired: 10 in]
        n204 = Bundle("分支"=enum16{"open", "read", "write", "close"}."write", "连接的字符串"=w365) -> (w364:T12)  [unwired: 1 in]
        n205 = Enqueue Element(queue=w369, element=w364, error in (no error)=w368) -> (queue out=w363:refnum<queue>, error out=w362:errorcluster)  [unwired: 1 in, 1 out]
        n206 = Enqueue Element(queue=w363, element=T5 {"分支"=enum."read", "字符串"=""} ("元素"), error in (no error)=w362) -> ()  [unwired: 1 in, 3 out]
      }
      event "查看型号": Value Change {
        n207 = event-data() -> ()  [unwired: 1 in, 6 out]
        n208 = One Button Dialog(message="空调品牌为:黑盾" ("消息")) -> ()  [unwired: 1 in, 1 out]
      }
    }
  }
